vi "data_download_single.vi"(8 "文件路径（使用对话框）":path, 10 "数值":dbl) -> ()   [LabVIEW 2020]
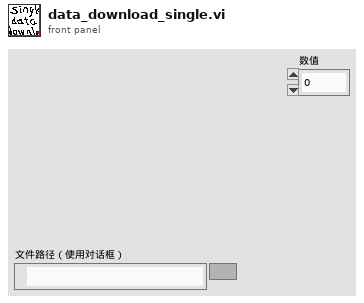
[diagram p1: front panel]
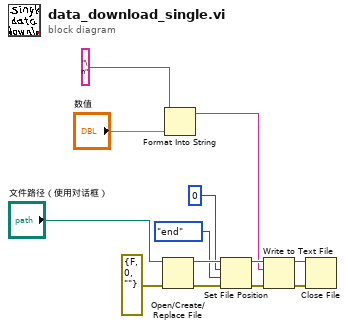
[diagram p0: block diagram]
diagram:
  n1 = Open/Create/Replace File(file path (use dialog)="文件路径（使用对话框）", error in=errorcluster {"status"=FALSE, "code"=0, "source"=""} ("错误输入")) -> (refnum out=w10:refnum<file>, error out=w12:errorcluster)  [unwired: 4 in, 1 out]
  n2 = Format Into String(initial string="\n" ("初始字符串"), "数值") -> (resulting string=w6:string)  [unwired: 2 in, 1 out]
  n3 = Set File Position(offset (in bytes) (0)=i64 0 ("偏移量（字节）（0）"), refnum=w10, from (0:start)=enum16{"start", "end", "current"}."end" ("自（0:起始）"), error in=w12) -> (refnum out=w9:refnum<file>, error out=w11:errorcluster)
  n4 = Write to Text File(file (use dialog)=w9, text=w6, error in=w11) -> (refnum out=w5:refnum<file>, error out=w4:errorcluster)  [unwired: 1 in, 1 out]
  n5 = Close File(refnum=w5, error in=w4) -> ()  [unwired: 2 out]
